vi "Welcome.vi"() -> ()   [LabVIEW 2017]
uses:
  Global/Global 1.vi
  Global/Login Details.vi
  Global/DATA LOG.vi
  Control/WELCOM SCREEN ENUM.ctl
panel:
  out "Screen Index":i32
  in  "Check 2":bool
  in  "auto":bool
  in  "Test Print":bool
  in  "andon":bool
  in  "MANUAL":bool
  out "error out 2":errorcluster
  in  "error in (no error) 3":errorcluster
  in  "Remove":bool
  in  "Check":bool
  in  "Home":bool
  out "user name":string
  out "STOP":bool
  in  "Tab Control":enum32{"Page 1", "user mangement"}(tab)
  out "error out":errorcluster
  in  "error in (no error)":errorcluster
  in  "LOGIN":bool
  in  "RECIPE":bool
  in  "EXIT":bool
  in  "REPORT":bool
  in  "Hardware Setting":bool
  in  "Shift Setting":bool
  in  "AUTO MODE":bool
  in  "USER MANGMENT":bool
  out "datetime":string
  # "PV Clean Mobility Technologies Traceability System"
  # "USER :"
  # "Powered By - NiVision Automation Systems Pvt. Ltd."
  # "Powered By-Infinity Automation Systems Pvt Ltd. Pune"
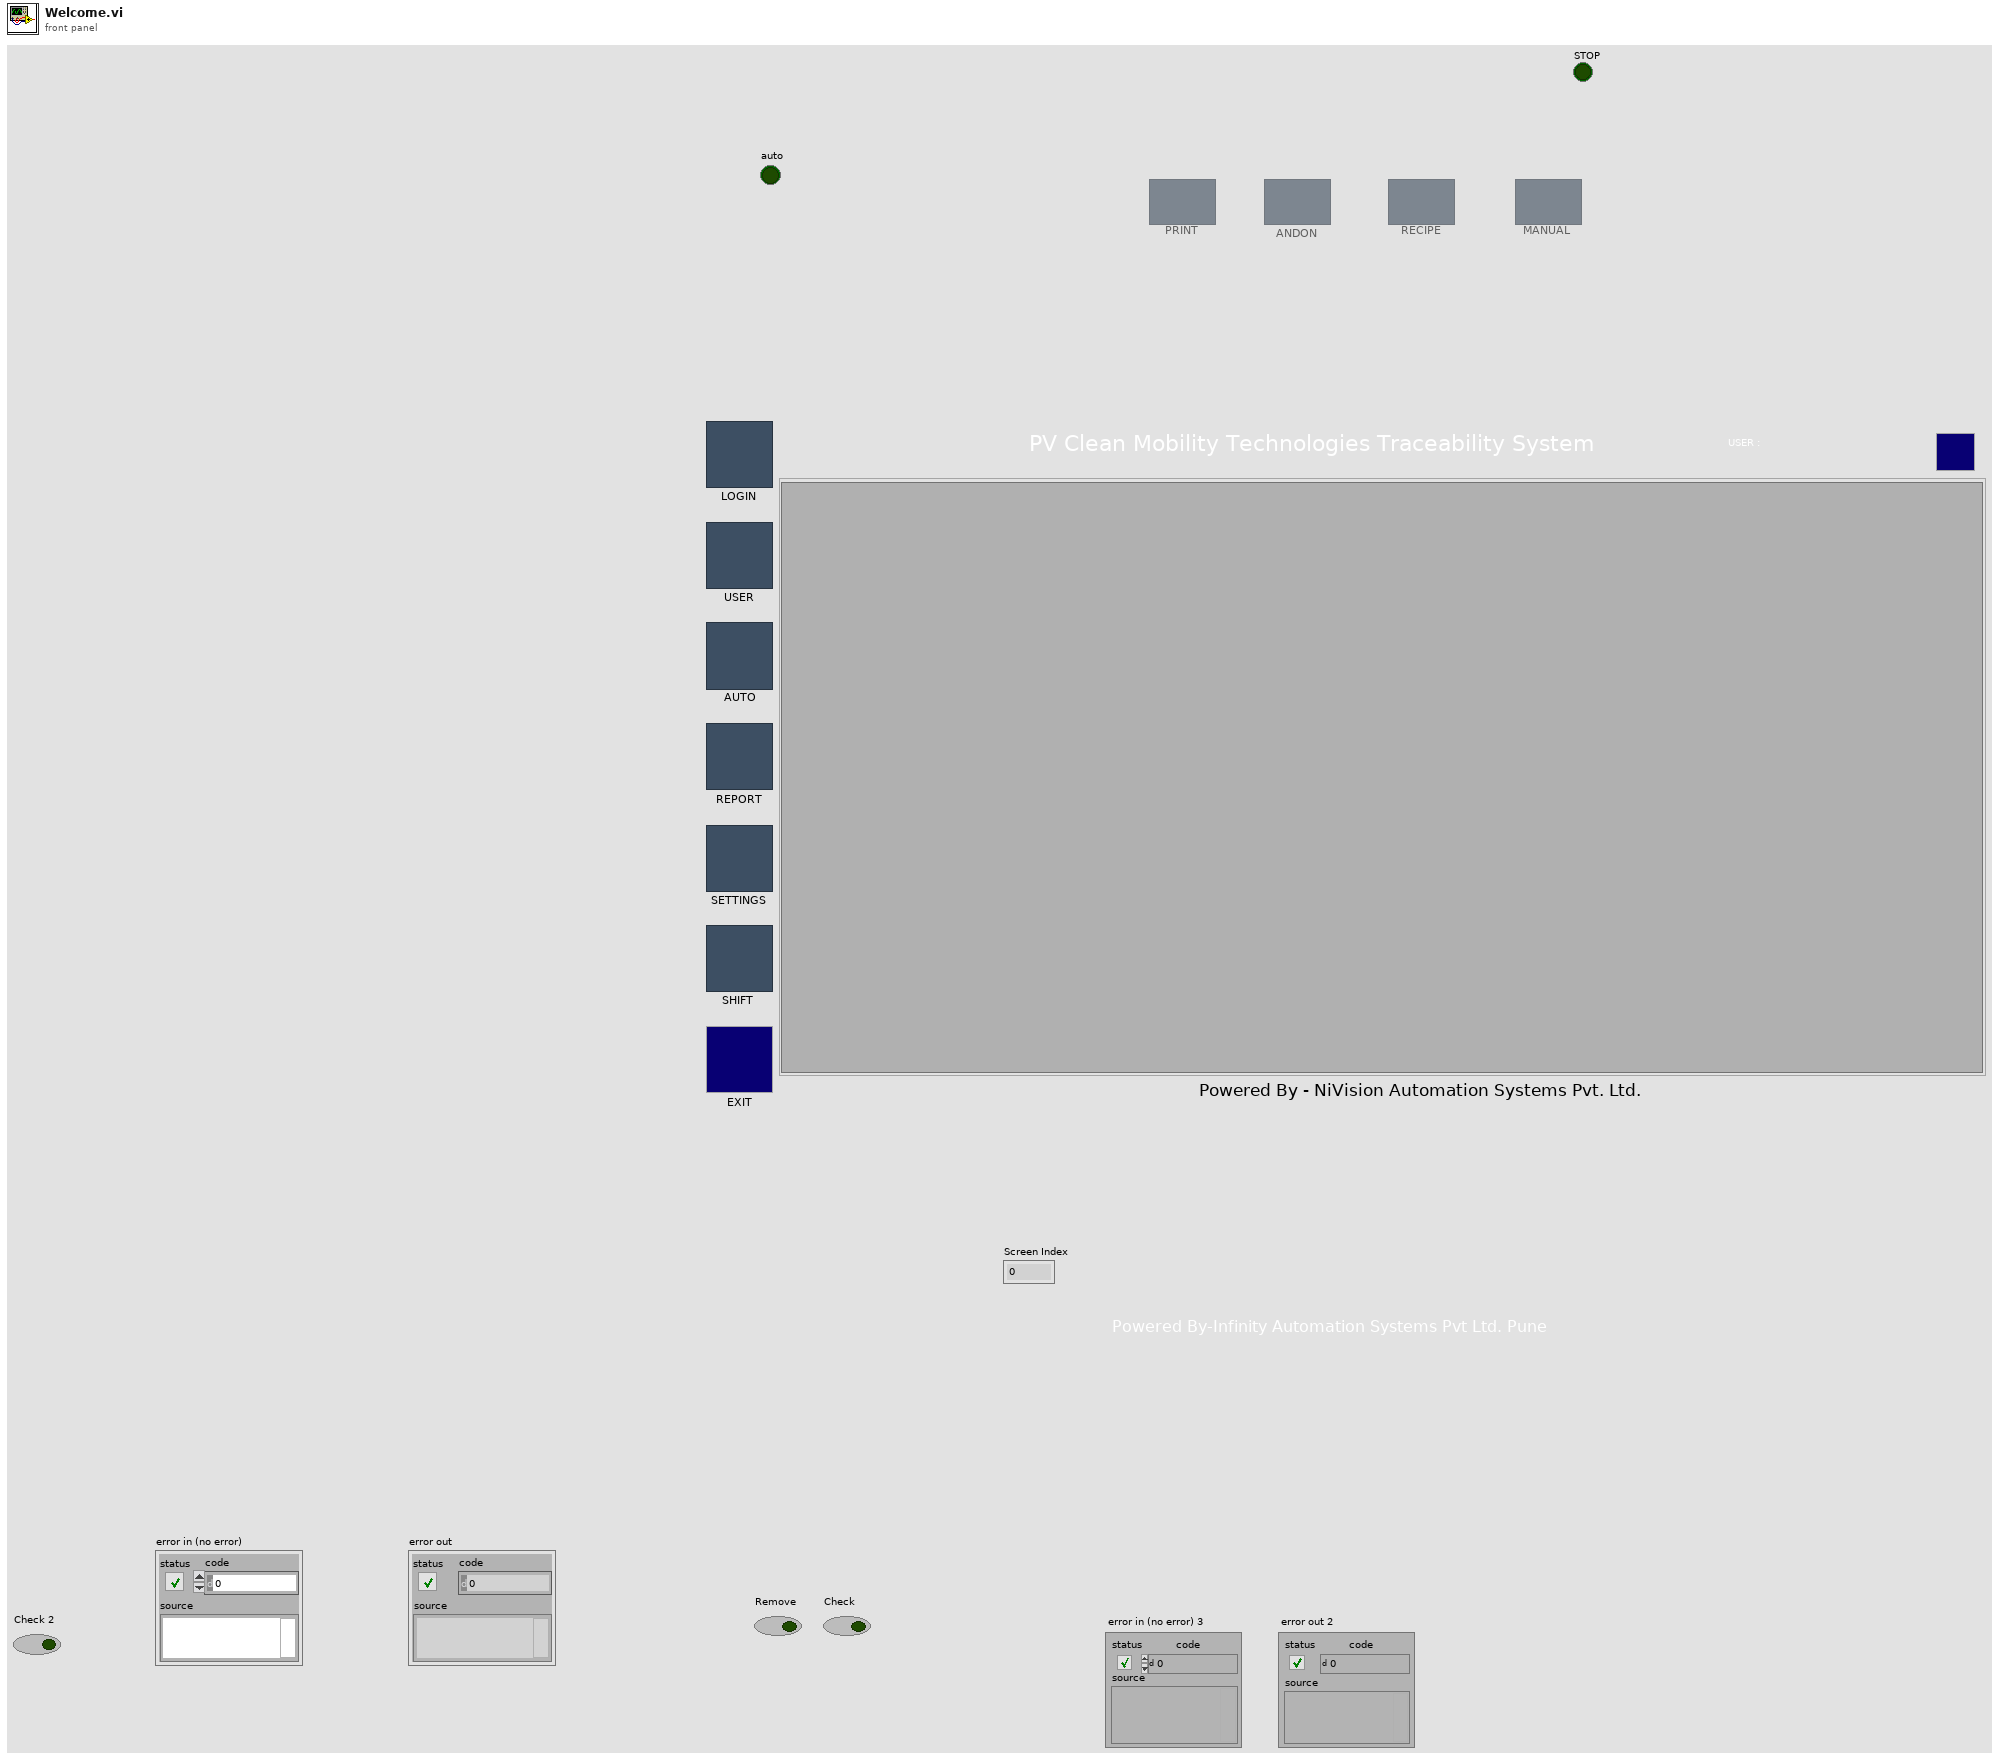
[diagram p1: front panel]
types:
  T1 = typedef "WELCOM SCREEN ENUM.ctl" = enum16{"Initialization", "Wait For Event", "RUN", "LOGIN", "USER MANAGEMENT", "AUTORITY MANAGEMENT", "AUTO MODE", "MANUAL MODE", "BIN MASTER", "CHEMICAL MASTER", "RAW MATERIAL INWARD", "RECIPE INGREDIENT", "REPORT", "SHIFT SETTING", "HARDWARE SETTING", "Check Authority", "TEST PRINT", "EXIT"}
  T2 = cluster{"SCREEN 1":bool, "SCREEN 2":bool, "SCREEN 3":bool, "SCREEN 4":bool, "SCREEN 5":bool, "SCREEN 6":bool, "SCREEN 7":bool, "SCREEN 8":bool, "SCREEN 9":bool, "SCREEN 10":bool, "SCREEN 11":bool, "SCREEN 12":bool, "SCREEN 13":bool, "SCREEN 14":bool, "SCREEN 15":bool, "SCREEN 16":bool, "SCREEN 17":bool, "SCREEN 18":bool, "SCREEN 19":bool, "SCREEN 20":bool}
  T3 = enum8{"Enabled", "Disabled", "Disabled and Grayed Out"}
  T4 = enum32{"Invalid", "Standard", "Closed", "Hidden", "Minimized", "Maximized"}
  T5 = enum32{"Bad", "Idle", "Run top level", "Running"}
  T6 = enum32{"invalid app kind", "Development System", "Run Time System", "Student Edition", "Embedded LabVIEW", "Evaluation", "Custom"}
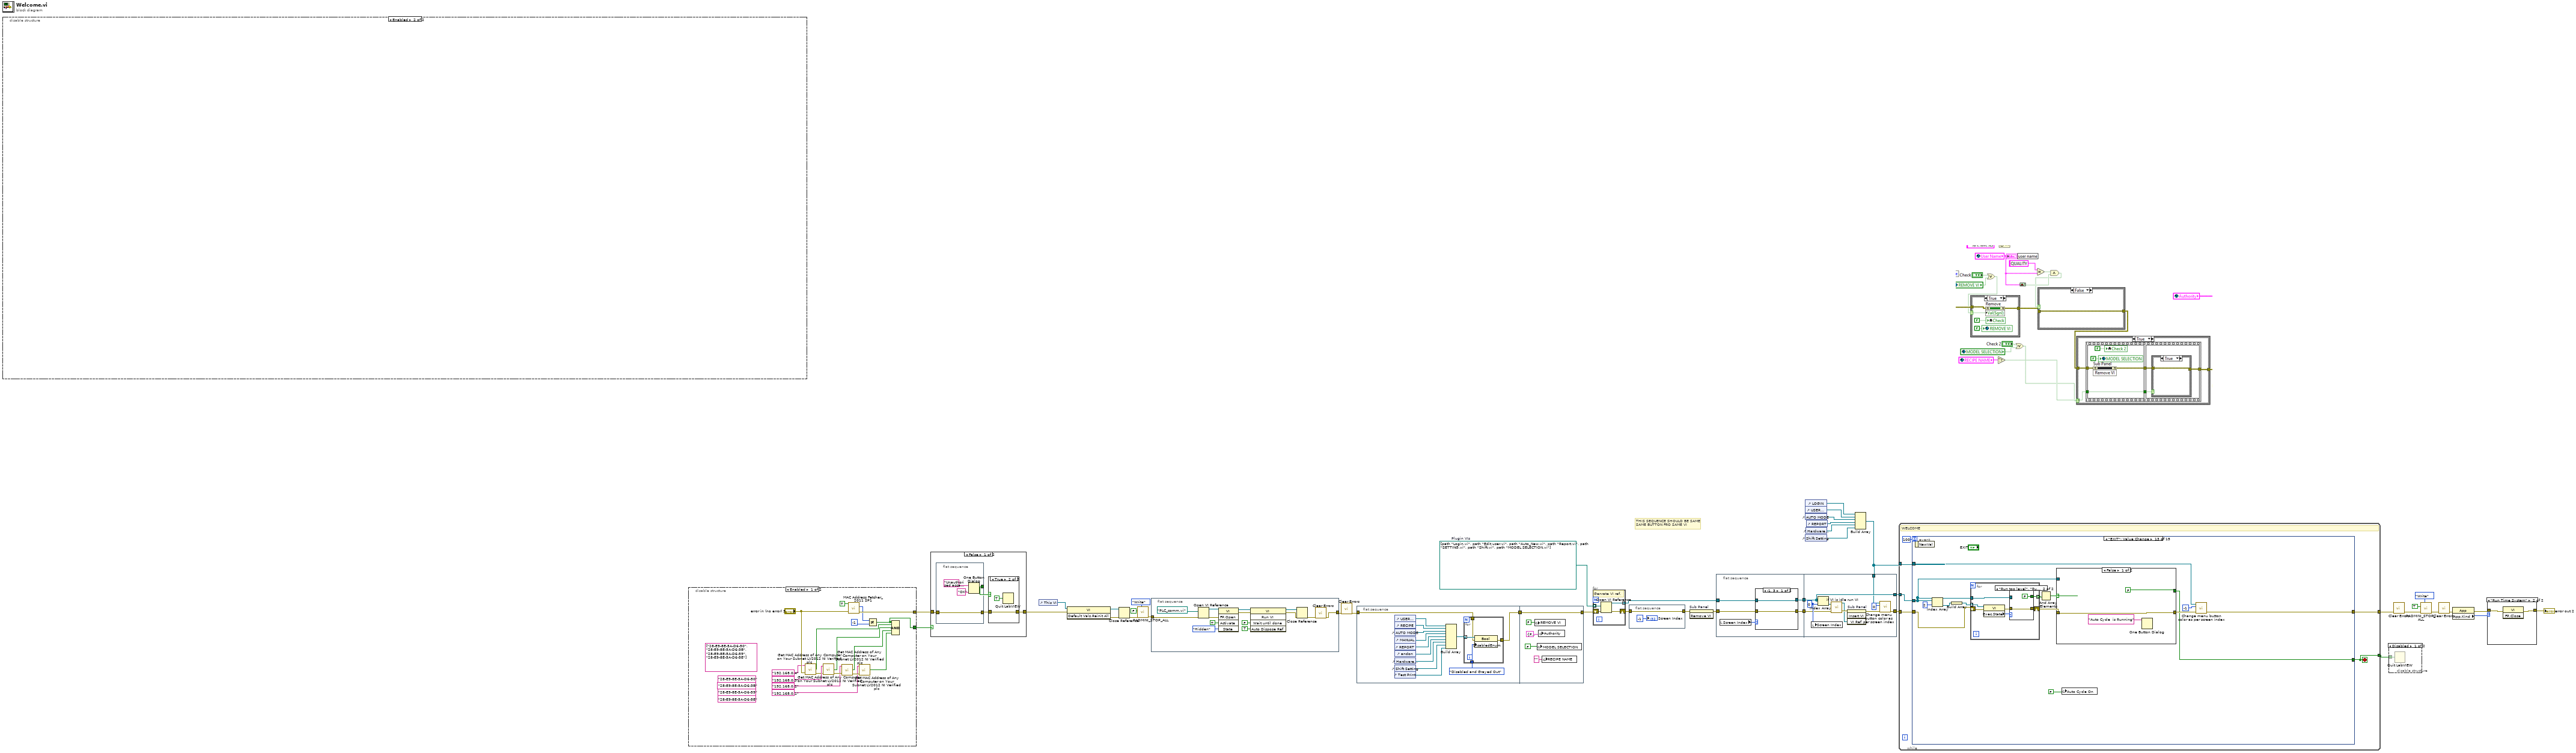
[diagram p0: block diagram]
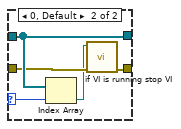
[diagram p2: hidden frame]
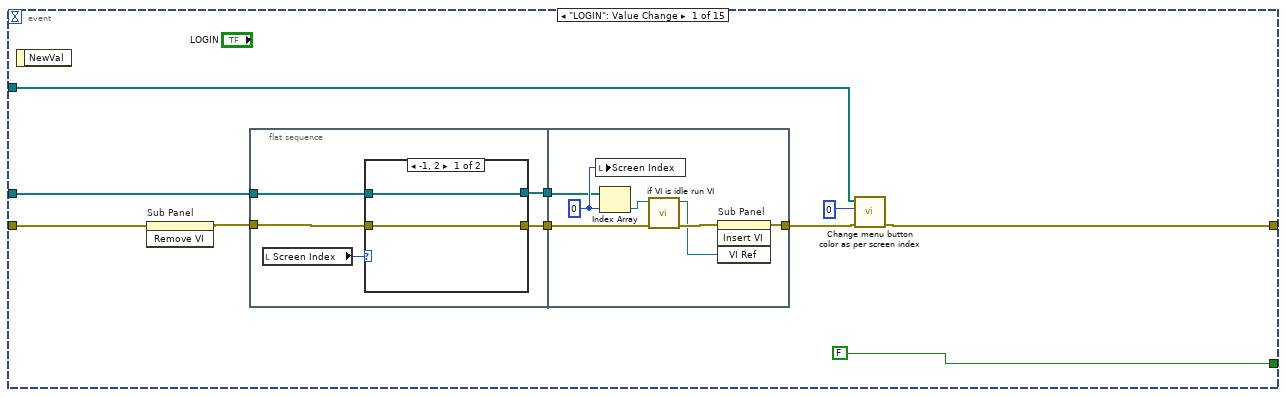
[diagram p5: hidden frame]
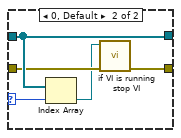
[diagram p6: hidden frame]
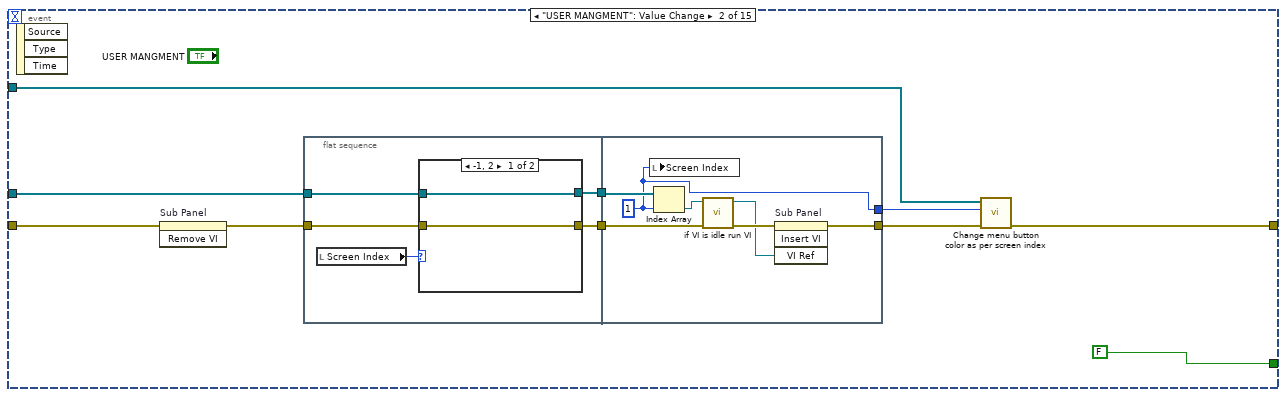
[diagram p7: hidden frame]
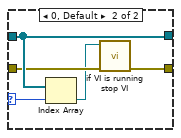
[diagram p8: hidden frame]
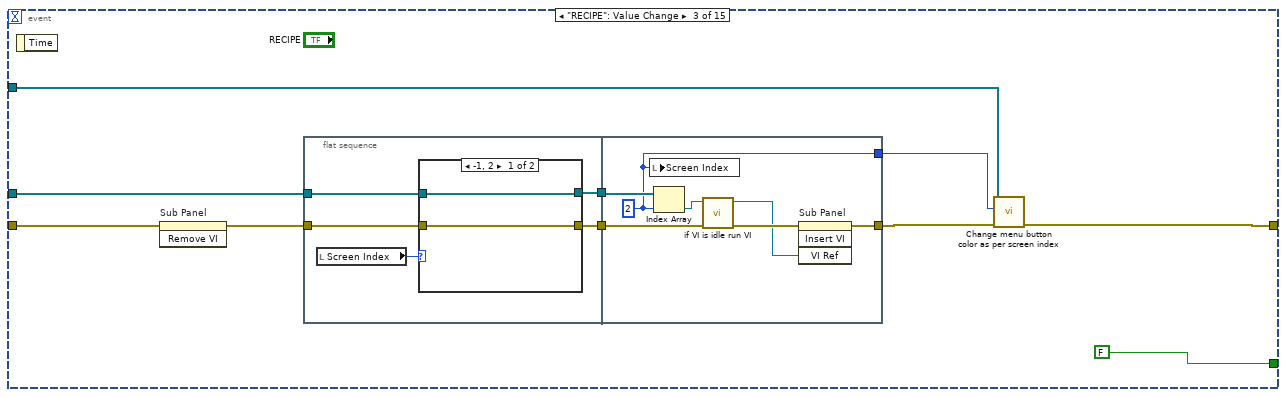
[diagram p9: hidden frame]
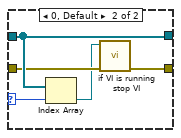
[diagram p10: hidden frame]
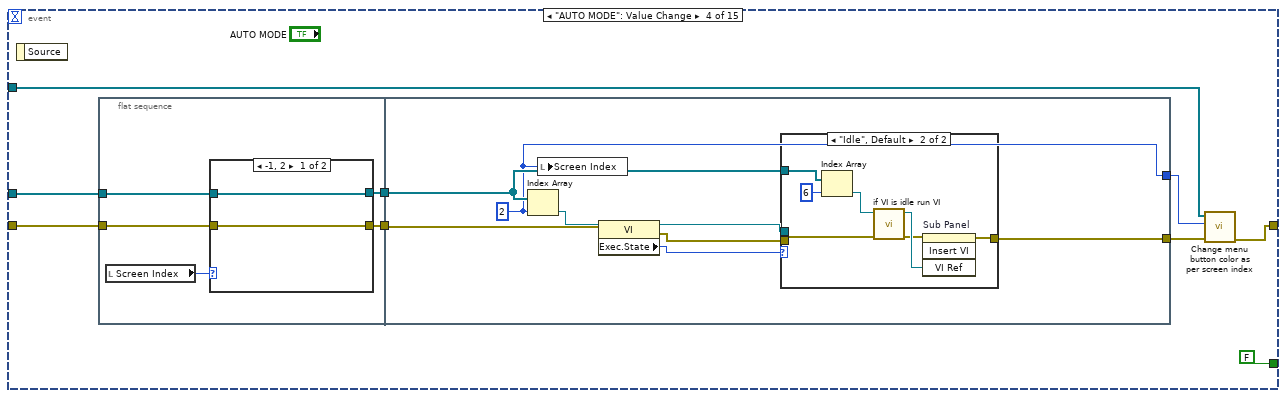
[diagram p11: hidden frame]
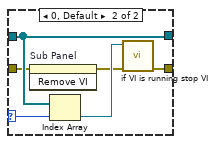
[diagram p12: hidden frame]
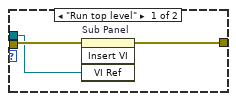
[diagram p13: hidden frame]
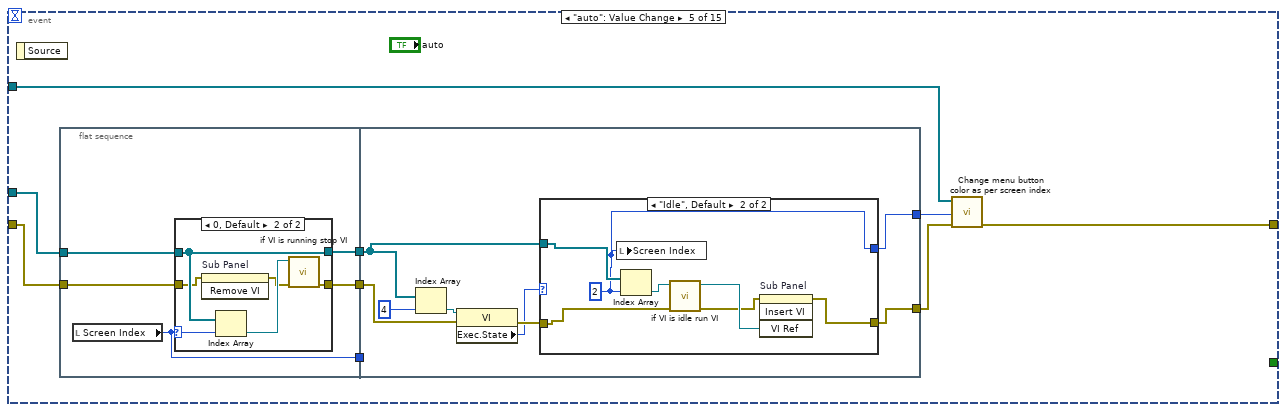
[diagram p14: hidden frame]
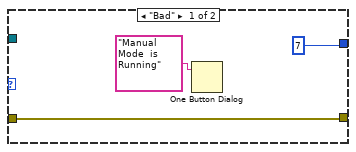
[diagram p16: hidden frame]
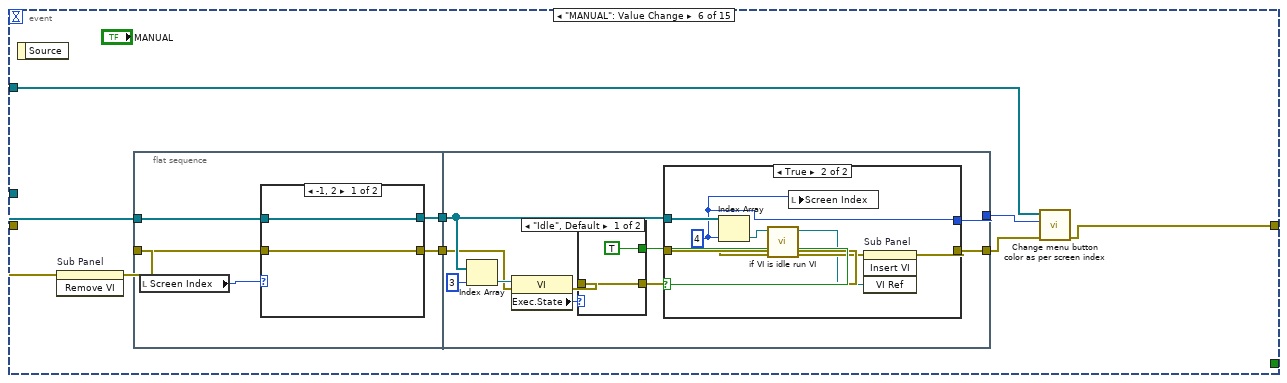
[diagram p17: hidden frame]
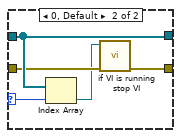
[diagram p18: hidden frame]
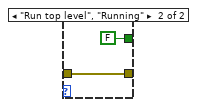
[diagram p19: hidden frame]
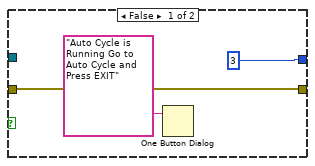
[diagram p20: hidden frame]
diagram:
  w33 = path[] [path "Login.vi", path "Edit user.vi", path "Auto_New.vi", path "Report.vi", path "SETTING.vi", path "Shift.vi", path "MODEL SELECTION.vi"]  # Plugin VIs
  # "THIS SEQUENCE SHOULD BE SAME\nSAME BUTTON FRO SAME VI"
  # "THIS SEQUENCE SHOULD BE SAME\nSAME BUTTON FRO SAME VI"
  n1 = disable-structure shown="Enabled" {
    frame Disabled {
      n2 = flat-sequence {
        tunnel: "error in (no error)" -> [w68]
        tunnel: [w67] -> w43
        frame #0 {
          n3 = invoke class="VI" method="Default Vals.Reinit All"(error in=w68) -> (error out=w67:errorcluster)  [unwired: 2 in, 2 out]
          n4 = global write "Login Details.vi" "Authority"(T2 {"SCREEN 1"=FALSE, "SCREEN 2"=FALSE, "SCREEN 3"=FALSE, "SCREEN 4"=FALSE, "SCREEN 5"=FALSE, "SCREEN 6"=FALSE, "SCREEN 7"=FALSE, "SCREEN 8"=FALSE, "SCREEN 9"=FALSE, "SCREEN 10"=FALSE, "SCREEN 11"=FALSE, "SCREEN 12"=FALSE, "SCREEN 13"=FALSE, "SCREEN 14"=FALSE, "SCREEN 15"=FALSE, "SCREEN 16"=FALSE, "SCREEN 17"=FALSE, "SCREEN 18"=FALSE, "SCREEN 19"=FALSE, "SCREEN 20"=FALSE} ("Authority")) -> ()
        }
      }
      n5 = invoke on="Sub Panel" class="SubPnl" method="Remove VI"(error in=w43) -> (error out=w56:errorcluster)  [unwired: 2 in, 2 out]
      n6 = Open VI Reference(vi path=path "Login.vi", error in (no error)=w56) -> (vi reference=w55:refnum<vi>, error out=w53:errorcluster)  [unwired: 4 in]
      n7 = invoke on="Sub Panel" class="SubPnl" method="Insert VI"(error in=w53, "VI Ref"=w55) -> (error out=w54:errorcluster)  [unwired: 2 in, 3 out]
      n8 = invoke class="VI" method="Run VI"(reference=w55, error in=w54, "Wait until done"=TRUE ("Wait Until Done"), "Auto Dispose Ref"=FALSE ("Auto Dispose Reference")) -> (reference out=w51:refnum<vi>, error out=w52:errorcluster)  [unwired: 1 in, 3 out]
      n9 = Close Reference(reference=w51, error in (no error)=w52) -> (error out=w46:errorcluster)
      n10 = Unbundle By Name(w46) -> ("code"=w50:i32)
      n11 = call <vilib>:"Clear Errors.vi"("error in (no error)"=w46) -> ("error out"=w48:errorcluster)  [unwired: 5 in, 1 out]
      n12 = Not Equal?(x=7, y=w50) -> (x != y?=w49:bool)
      n13 = Select(t=w46, s=w49, f=w48) -> (s? t:f=w47:errorcluster)
      n14 = call <vilib>:"Simple Error Handler.vi"("error in (no error)"=w47) -> ("error out"=w57:errorcluster)  [unwired: 4 in, 4 out]
      n15 = invoke on="Sub Panel" class="SubPnl" method="Remove VI"(error in=w57) -> (error out=w45:errorcluster)  [unwired: 2 in, 2 out]
      n16 = while {
        tunnel: w45 -> [w75]
        shift-right: [w77] -> _
        shift-left: WELCOM_SCREEN_ENUM."Initialization" -> [w71]
        shift-right: [w74] -> _
        shift-left: cluster{"VI Run":string} {"VI Run"=""} -> [w73]
        tunnel: [w76] -> w63
        stop <- w72 stop-if-true
        n17 = case shown="\"AUTORITY MANAGEMENT\"" w71 {
          tunnel: [WELCOM_SCREEN_ENUM."Check Authority" w102 WELCOM_SCREEN_ENUM."Wait For Event" WELCOM_SCREEN_ENUM."Wait For Event" WELCOM_SCREEN_ENUM."RUN" WELCOM_SCREEN_ENUM."RUN" WELCOM_SCREEN_ENUM."RUN" WELCOM_SCREEN_ENUM."RUN" WELCOM_SCREEN_ENUM."RUN" WELCOM_SCREEN_ENUM."RUN" WELCOM_SCREEN_ENUM."RUN" WELCOM_SCREEN_ENUM."RUN" WELCOM_SCREEN_ENUM."RUN" WELCOM_SCREEN_ENUM."RUN" WELCOM_SCREEN_ENUM."RUN" WELCOM_SCREEN_ENUM."RUN" WELCOM_SCREEN_ENUM."RUN" w229] -> w77
          tunnel: [w95 w101 w123 w127 w133 w139 w145 w151 w157 w163 w169 w175 w181 w187 w193 w199 w205 w224] -> w76
          tunnel: w75 -> [w95 w101 w123 w127 w133 w139 w145 w151 w157 w163 w169 w175 w181 w187 w193 w199 w205 w223]
          tunnel: [w93 w99 w122 w126 w131 w137 w142 w146 w155 w161 w167 w170 w177 w185 w188 w194 w203 w222] -> w74
          tunnel: w73 -> [w93 w99 w122 w126 w132 w138 w143 w147 w156 w162 w168 w171 w178 w186 w189 w195 w204 w222]
          tunnel: [FALSE FALSE FALSE TRUE FALSE FALSE FALSE FALSE FALSE FALSE FALSE FALSE FALSE FALSE FALSE FALSE FALSE FALSE] -> w72
          frame "Initialization", Default {
            n18 = control-ref of="USER MANGMENT"() -> (w80:refnum<vi>)
            n19 = control-ref of="RECIPE"() -> (w81:refnum<vi>)
            n20 = control-ref of="AUTO MODE"() -> (w82:refnum<vi>)
            n21 = control-ref of="REPORT"() -> (w88:refnum<vi>)
            n22 = control-ref of="Shift Setting"() -> (w89:refnum<vi>)
            n23 = control-ref of="Hardware Setting"() -> (w90:refnum<vi>)
            n24 = Build Array(w80, w81, w82, w88, w89, w90) -> (w79:refnum<vi>[], w83:refnum<vi>, w84:refnum<vi>, w85:refnum<vi>, w86:refnum<vi>, w87:refnum<vi>, w91:refnum<vi>)
            n25 = for {
              tunnel: w79 -> [w97] mode=indexing
              n26 = property class="Bool"(reference=w97, "DisabledEnum"=T3."Disabled and Grayed Out" ("Disabled")) -> ()  [unwired: 1 in, 2 out]
            }
          }
          frame "Wait For Event" {
            n27 = Search 1D Array(1D array=bool[] [], element=TRUE) -> (index of element=w104:i32)  [unwired: 1 in]
            n28 = case shown="11" w104 {
              tunnel: [WELCOM_SCREEN_ENUM."Wait For Event" WELCOM_SCREEN_ENUM."EXIT" WELCOM_SCREEN_ENUM."LOGIN" WELCOM_SCREEN_ENUM."USER MANAGEMENT" WELCOM_SCREEN_ENUM."AUTORITY MANAGEMENT" WELCOM_SCREEN_ENUM."AUTO MODE" WELCOM_SCREEN_ENUM."MANUAL MODE" WELCOM_SCREEN_ENUM."BIN MASTER" WELCOM_SCREEN_ENUM."CHEMICAL MASTER" WELCOM_SCREEN_ENUM."RAW MATERIAL INWARD" WELCOM_SCREEN_ENUM."REPORT" WELCOM_SCREEN_ENUM."SHIFT SETTING" WELCOM_SCREEN_ENUM."HARDWARE SETTING" WELCOM_SCREEN_ENUM."TEST PRINT" WELCOM_SCREEN_ENUM."RECIPE INGREDIENT"] -> w102
              frame -1, Default {
              }
              frame 0 {
              }
              frame 1 {
              }
              frame 2 {
              }
              frame 3 {
              }
              frame 4 {
              }
              frame 5 {
              }
              frame 6 {
              }
              frame 7 {
              }
              frame 8 {
              }
              frame 9 {
              }
              frame 10 {
              }
              frame 11 {
              }
              frame 12 {
              }
              frame 13 {
              }
            }
          }
          frame "Check Authority" {
          }
          frame "EXIT" {
          }
          frame "LOGIN" {
            w130 = "Login.vi"  # VI Run
            n29 = Bundle By Name(cluster=w132, "VI Run"=w130) -> (w131:cluster{"VI Run":string})
          }
          frame "USER MANAGEMENT" {
            w136 = "User Management.vi"  # VI Run
            n30 = Bundle By Name(cluster=w138, "VI Run"=w136) -> (w137:cluster{"VI Run":string})
          }
          frame "AUTORITY MANAGEMENT" {
            w141 = "Authority Management.vi"  # VI Run
            n31 = Bundle By Name(cluster=w143, "VI Run"=w141) -> (w142:cluster{"VI Run":string})
          }
          frame "AUTO MODE" {
            w148 = "AUTO MODE.vi"  # VI Run
            n32 = Bundle By Name(cluster=w147, "VI Run"=w148) -> (w146:cluster{"VI Run":string})
          }
          frame "MANUAL MODE" {
            w154 = "Manual Mode.vi"  # VI Run
            n33 = Bundle By Name(cluster=w156, "VI Run"=w154) -> (w155:cluster{"VI Run":string})
          }
          frame "BIN MASTER" {
            w160 = "Bin Master.vi"  # VI Run
            n34 = Bundle By Name(cluster=w162, "VI Run"=w160) -> (w161:cluster{"VI Run":string})
          }
          frame "CHEMICAL MASTER" {
            w166 = "Chemical Master.vi"  # VI Run
            n35 = Bundle By Name(cluster=w168, "VI Run"=w166) -> (w167:cluster{"VI Run":string})
          }
          frame "RAW MATERIAL INWARD" {
            w172 = "raw material inward.vi"  # VI Run
            n36 = Bundle By Name(cluster=w171, "VI Run"=w172) -> (w170:cluster{"VI Run":string})
          }
          frame "RECIPE INGREDIENT" {
            w179 = "Recipe_Ingredients.vi"  # VI Run
            n37 = Bundle By Name(cluster=w178, "VI Run"=w179) -> (w177:cluster{"VI Run":string})
          }
          frame "REPORT" {
            w184 = "Report.vi"  # VI Run
            n38 = Bundle By Name(cluster=w186, "VI Run"=w184) -> (w185:cluster{"VI Run":string})
          }
          frame "SHIFT SETTING" {
            w190 = "shift setting.vi"  # VI Run
            n39 = Bundle By Name(cluster=w189, "VI Run"=w190) -> (w188:cluster{"VI Run":string})
          }
          frame "HARDWARE SETTING" {
            w196 = "Hardware Setting.vi"  # VI Run
            n40 = Bundle By Name(cluster=w195, "VI Run"=w196) -> (w194:cluster{"VI Run":string})
          }
          frame "TEST PRINT" {
            w202 = "Test Print.vi"  # VI Run
            n41 = Bundle By Name(cluster=w204, "VI Run"=w202) -> (w203:cluster{"VI Run":string})
          }
          frame "RUN" {
            w230 = "Login.vi"  # x
            n42 = Unbundle By Name(w222) -> ("VI Run"=w231:string)
            n43 = invoke on="Sub Panel" class="SubPnl" method="Remove VI"(error in=w223) -> (error out=w212:errorcluster)  [unwired: 2 in, 2 out]
            n44 = Equal?(x=w230, y=w231) -> (x = y?=w228:bool)
            n45 = String To Path(string=w231) -> (path=w207:path)
            n46 = Open VI Reference(vi path=w207, error in (no error)=w212) -> (vi reference=w213:refnum<vi>, error out=w215:errorcluster)  [unwired: 4 in]
            n47 = invoke on="Sub Panel" class="SubPnl" method="Insert VI"(error in=w215, "VI Ref"=w213) -> (error out=w214:errorcluster)  [unwired: 2 in, 3 out]
            n48 = invoke class="VI" method="Run VI"(reference=w213, error in=w214, "Wait until done"=TRUE ("Wait Until Done"), "Auto Dispose Ref"=FALSE ("Auto Dispose Reference")) -> (reference out=w217:refnum<vi>, error out=w216:errorcluster)  [unwired: 1 in, 3 out]
            n49 = Close Reference(reference=w217, error in (no error)=w216) -> (error out=w206:errorcluster)
            n50 = Unbundle By Name(w206) -> ("code"=w218:i32)
            n51 = call <vilib>:"Clear Errors.vi"("error in (no error)"=w206) -> ("error out"=w220:errorcluster)  [unwired: 5 in, 1 out]
            n52 = Not Equal?(x=7, y=w218) -> (x != y?=w219:bool)
            n53 = Select(t=WELCOM_SCREEN_ENUM."Check Authority", s=w228, f=WELCOM_SCREEN_ENUM."Wait For Event") -> (s? t:f=w229:T1)
            n54 = Select(t=w206, s=w219, f=w220) -> (s? t:f=w221:errorcluster)
            n55 = call <vilib>:"Simple Error Handler.vi"("error in (no error)"=w221) -> ("error out"=w211:errorcluster)  [unwired: 4 in, 4 out]
            n56 = invoke on="Sub Panel" class="SubPnl" method="Remove VI"(error in=w211) -> (error out=w224:errorcluster)  [unwired: 2 in, 2 out]
          }
        }
        "STOP" <- w72
        n57 = Wait (ms)(milliseconds to wait=u32 100) -> ()  [unwired: 1 out]
      }
      n58 = while {
        tunnel: w43 -> [w65]
        tunnel: [w65] -> w41
        stop <- w66 stop-if-true
        n59 = local read "STOP"() -> (w66:bool)
      }
      n60 = Merge Errors(w41, w63) -> (→"error out":errorcluster)
      n61 = disable-structure shown="Enabled" {
        disable-tunnel: w63 -> [w70 _]
        frame Enabled {
          n62 = invoke class="VI" method="FP.Close"(error in=w70) -> ()  [unwired: 2 in, 3 out]
        }
        frame Disabled {
        }
      }
    }
    frame Enabled {
    }
  }
  n63 = disable-structure shown="Enabled" {
    disable-tunnel: [w247 _] -> w5
    disable-tunnel: [w232 TRUE] -> w1
    frame Enabled {
      (unwired) string[] ["28-E9-8E-5A-D6-50", "28-E9-8E-5A-D6-3B", "28-E9-8E-5A-D6-59", "28-E9-8E-5A-D6-5E"]
      (unwired) "28-E9-8E-5A-D6-5E" ("IP Address")
      (unwired) "28-E9-8E-5A-D6-59" ("IP Address")
      (unwired) "28-E9-8E-5A-D6-3B" ("IP Address")
      (unwired) "28-E9-8E-5A-D6-50" ("IP Address")
      n64 = call "Get MAC Address of Any Computer on Your Subnet LV2012 NI Verified plc.vi"("error constant"="error in (no error) 3", "IP Address"="192.168.0.4") -> ("error out"=w243:errorcluster, "x .and. y?"=w236:bool)  [unwired: 1 in, 1 out]
      n65 = call "Get MAC Address of Any Computer on Your Subnet LV2012 NI Verified plc.vi"("error constant"=w243, "IP Address"="192.168.0.3") -> ("error out"=w241:errorcluster, "x .and. y?"=w235:bool)  [unwired: 1 in, 1 out]
      n66 = call "Get MAC Address of Any Computer on Your Subnet LV2012 NI Verified plc.vi"("error constant"=w241, "IP Address"="192.168.0.2") -> ("error out"=w242:errorcluster, "x .and. y?"=w234:bool)  [unwired: 1 in, 1 out]
      n67 = call "MAC Address Fetcher_2011 SP1.vi"("error in (no error)"="error in (no error) 3", "Search all adapters?"=TRUE) -> ("error out"=w247:errorcluster, "index of element"=w238:i32)  [unwired: 6 in, 2 out]
      n68 = call "Get MAC Address of Any Computer on Your Subnet LV2012 NI Verified plc.vi"("error constant"=w242, "IP Address"="192.168.0.1") -> ("x .and. y?"=w233:bool)  [unwired: 1 in, 2 out]
      n69 = Not Equal?(x=w238, y=-1) -> (x != y?=w232:bool)
      n70 = Compound Arithmetic op=AND(w232, w236, w235, w234, w233) -> ()  [unwired: 1 out]
    }
    frame Disabled {
    }
  }
  n71 = case shown="False" w1 {
    tunnel: w5 -> [w251 w261]
    tunnel: [w250 w261] -> w4
    frame False {
      n72 = flat-sequence {
        tunnel: [w256] -> w253
        tunnel: [w255] -> w252
        tunnel: w251 -> [w255]
        frame #0 {
          n73 = One Button Dialog(message="Unauthorised access to this system\nPlease contact to NIVision Automation Systems Pvt Ltd", button name ("OK")="OK") -> (true=w256:bool)
        }
      }
      n74 = case shown="True" w253 {
        tunnel: w252 -> [w258 w259]
        tunnel: [w258 w259] -> w250
        frame False {
        }
        frame True {
          n75 = Quit LabVIEW(quit? (T)=TRUE) -> ()
        }
      }
    }
    frame True {
    }
  }
  n76 = control-ref of="This VI"() -> (w40:refnum<vi>)
  n77 = invoke class="VI" method="Default Vals.Reinit All"(reference=w40, error in=w4) -> (reference out=w38:refnum<vi>, error out=w39:errorcluster)  [unwired: 1 in, 1 out]
  n78 = Close Reference(reference=w38, error in (no error)=w39) -> (error out=w2:errorcluster)
  n79 = call "PADMINI_STOP_ALL.vi"("Enum"=enum16{"Read", "Write"}."Write", "error in (no error)"=w2, "Boolean"=FALSE) -> ("error out"=w6:errorcluster)  [unwired: 7 in, 1 out]
  n80 = flat-sequence {
    tunnel: w6 -> [w275]
    tunnel: [w273] -> w21
    frame #0 {
      n81 = Open VI Reference(vi path=path "PLC_comm.vi", error in (no error)=w275) -> (vi reference=w266:refnum<vi>, error out=w267:errorcluster)  [unwired: 4 in]
      n82 = invoke class="VI" method="FP.Open"(reference=w266, error in=w267, "Activate"=TRUE ("Activate?"), "State"=T4."Hidden") -> (reference out=w269:refnum<vi>, error out=w268:errorcluster)  [unwired: 1 in, 3 out]
      n83 = invoke class="VI" method="Run VI"(reference=w269, error in=w268, "Wait until done"=FALSE ("Wait Until Done"), "Auto Dispose Ref"=TRUE ("Auto Dispose Reference")) -> (reference out=w264:refnum<vi>, error out=w263:errorcluster)  [unwired: 1 in, 3 out]
      n84 = Close Reference(reference=w264, error in (no error)=w263) -> (error out=w274:errorcluster)
      n85 = call <vilib>:"Clear Errors.vi"("error in (no error)"=w274) -> ("error out"=w273:errorcluster)  [unwired: 5 in, 1 out]
    }
  }
  n86 = call <vilib>:"Clear Errors.vi"("error in (no error)"=w21) -> ("error out"=w20:errorcluster)  [unwired: 5 in, 1 out]
  n87 = flat-sequence {
    tunnel: w20 -> [w277]
    tunnel: [w276] -> w13
    tunnel: [w297] -> w23
    tunnel: w13 -> [w297]
    frame #0 {
      n88 = control-ref of="Shift Setting"() -> (w281:refnum<vi>)
      n89 = control-ref of="Test Print"() -> (w280:refnum<vi>)
      n90 = control-ref of="USER MANGMENT"() -> (w288:refnum<vi>)
      n91 = control-ref of="RECIPE"() -> (w287:refnum<vi>)
      n92 = control-ref of="AUTO MODE"() -> (w286:refnum<vi>)
      n93 = control-ref of="MANUAL"() -> (w285:refnum<vi>)
      n94 = control-ref of="REPORT"() -> (w284:refnum<vi>)
      n95 = control-ref of="andon"() -> (w283:refnum<vi>)
      n96 = control-ref of="Hardware Setting"() -> (w282:refnum<vi>)
      n97 = Build Array(w288, w287, w286, w285, w284, w283, w282, w281, w280) -> (w279:refnum<vi>[])
      n98 = for {
        tunnel: w279 -> [w292] mode=indexing
        tunnel: w277 -> [w291]
        tunnel: T3."Disabled and Grayed Out" ("Disabled") -> [w290]
        tunnel: [w289] -> w276
        n99 = property class="Bool"(reference=w292, error in=w291, "DisabledEnum"=w290) -> (error out=w289:errorcluster)  [unwired: 1 out]
      }
    }
    frame #1 {
      n100 = global write "Global 1.vi" "REMOVE VI"(FALSE ("REMOVE VI")) -> ()
      n101 = global write "Global 1.vi" "MODEL SELECTION"(FALSE ("REMOVE VI")) -> ()
      n102 = global write "Login Details.vi" "Authority"(T2 {"SCREEN 1"=FALSE, "SCREEN 2"=FALSE, "SCREEN 3"=FALSE, "SCREEN 4"=FALSE, "SCREEN 5"=FALSE, "SCREEN 6"=FALSE, "SCREEN 7"=FALSE, "SCREEN 8"=FALSE, "SCREEN 9"=FALSE, "SCREEN 10"=FALSE, "SCREEN 11"=FALSE, "SCREEN 12"=FALSE, "SCREEN 13"=FALSE, "SCREEN 14"=FALSE, "SCREEN 15"=FALSE, "SCREEN 16"=FALSE, "SCREEN 17"=FALSE, "SCREEN 18"=FALSE, "SCREEN 19"=FALSE, "SCREEN 20"=FALSE} ("Authority")) -> ()
      n103 = global write "Global 1.vi" "RECIPE NAME"("" ("RECIPE NAME")) -> ()
    }
  }
  n104 = for {
    tunnel: w33 -> [w299] mode=indexing
    tunnel: [w300] -> w26 mode=indexing
    shift-right: [w301] -> w32
    shift-left: w23 -> [w298]
    # "Genrate VI ref."
    n105 = Open VI Reference(vi path=w299, error in (no error)=w298) -> (vi reference=w300:refnum<vi>, error out=w301:errorcluster)  [unwired: 4 in]
  }
  n106 = flat-sequence {
    tunnel: w32 -> [w303]
    tunnel: [w303] -> w28
    frame #0 {
      "Screen Index" <- -1 ("Screen Index")
    }
  }
  n107 = invoke on="Sub Panel" class="SubPnl" method="Remove VI"(error in=w28) -> (error out=w29:errorcluster)  [unwired: 2 in, 2 out]
  n108 = flat-sequence {
    tunnel: w26 -> [w306]
    tunnel: [w308] -> w31
    tunnel: [w305] -> w30
    tunnel: w29 -> [w304]
    tunnel: w31 -> [w324]
    tunnel: w30 -> [w320]
    tunnel: [w317] -> w27
    tunnel: [w320] -> w25
    tunnel: w24 -> [w316]
    frame #0 {
      n109 = local read "Screen Index"() -> (w307:i32)
      n110 = case shown="-1, 3" w307 {
        selector: w307 -> [_ w315]
        tunnel: w304 -> [w310 w313]
        tunnel: [w310 w312] -> w308
        tunnel: w306 -> [w309 w314]
        tunnel: [w309 w314] -> w305
        frame -1, 3 {
        }
        frame 0, Default {
          n111 = Index Array(array=w314, index=w315) -> (element=w311:refnum<vi>)
          n112 = call "if VI is running stop VI.vi"("error in (no error)"=w313, "VI in"=w311) -> ("error out"=w312:errorcluster)  [unwired: 8 in, 1 out]
        }
      }
    }
    frame #1 {
      w325 = 0 ("index")
      n113 = local write "Screen Index"(w325) -> ()
      n114 = Index Array(array=w320, index=w325) -> (element=w323:refnum<vi>)
      n115 = call "if VI is idle run VI.vi"("error in (no error)"=w324, "VI in"=w323) -> ("error out"=w322:errorcluster, "VI out"=w321:refnum<vi>)  [unwired: 8 in]
      n116 = invoke on="Sub Panel" class="SubPnl" method="Insert VI"(error in=w322, "VI Ref"=w321) -> (error out=w318:errorcluster)  [unwired: 2 in, 3 out]
      n117 = call "Change menu button color as per screen index.vi"("error in (no error)"=w318, "Screen Index"=0, "Array"=w316) -> ("error out"=w317:errorcluster)  [unwired: 8 in]
    }
  }
  n118 = control-ref of="LOGIN"() -> (w19:refnum<vi>)
  n119 = control-ref of="USER MANGMENT"() -> (w18:refnum<vi>)
  n120 = control-ref of="AUTO MODE"() -> (w17:refnum<vi>)
  n121 = control-ref of="Shift Setting"() -> (w14:refnum<vi>)
  n122 = control-ref of="Hardware Setting"() -> (w15:refnum<vi>)
  n123 = control-ref of="REPORT"() -> (w16:refnum<vi>)
  n124 = Build Array(w19, w18, w17, w16, w15, w14) -> (w24:refnum<vi>[])
  n125 = while {
    tunnel: w27 -> [w328]
    tunnel: [w330] -> w22
    tunnel: w25 -> [w327]
    tunnel: w24 -> [w329]
    tunnel: [w326] -> w3
    stop <- w326 stop-if-true
    # "WELCOME"
    n126 = event shown="[12] \"EXIT\": Value Change" {
      selector: _ -> [_ _ _ _ _ _ _ _ _ _ _ _ _ _ _]
      dyn-events: _ -> [_ _ _ _ _ _ _ _ _ _ _ _ _ _ _]
      timeout: 100 -> [_ _ _ _ _ _ _ _ _ _ _ _ _ _ _]
      tunnel: [FALSE FALSE FALSE FALSE _ _ FALSE FALSE FALSE FALSE FALSE FALSE w697 FALSE FALSE] -> w326
      tunnel: [w334 w365 w394 w426 w459 w499 w548 w577 w606 w635 w664 w691 w696 w737 w740] -> w330
      tunnel: w327 -> [w340 w369 w398 w422 w463 w502 w552 w581 w610 w639 w668 _ w698 _ _]
      tunnel: w329 -> [w333 w363 w391 w425 w462 w500 w546 w574 w603 w633 w661 w690 w701 w735 _]
      tunnel: w328 -> [w332 w361 w390 w421 w464 w501 w544 w573 w602 w631 w660 w689 w705 w734 w752]
      event "LOGIN": Value Change {
        n127 = event-data() -> ()  [unwired: 1 in, 1 out]
        n128 = invoke on="Sub Panel" class="SubPnl" method="Remove VI"(error in=w332) -> (error out=w337:errorcluster)  [unwired: 2 in, 2 out]
        n129 = flat-sequence {
          tunnel: w340 -> [w344]
          tunnel: [w346] -> w339
          tunnel: [w343] -> w338
          tunnel: w337 -> [w342]
          tunnel: w339 -> [w358]
          tunnel: w338 -> [w359]
          tunnel: [w354] -> w335
          frame #0 {
            n130 = local read "Screen Index"() -> (w345:i32)
            n131 = case shown="-1, 2" w345 {
              selector: w345 -> [_ w353]
              tunnel: w342 -> [w348 w351]
              tunnel: [w348 w350] -> w346
              tunnel: w344 -> [w347 w352]
              tunnel: [w347 w352] -> w343
              frame -1, 2 {
              }
              frame 0, Default {
                n132 = Index Array(array=w352, index=w353) -> (element=w349:refnum<vi>)
                n133 = call "if VI is running stop VI.vi"("error in (no error)"=w351, "VI in"=w349) -> ("error out"=w350:errorcluster)  [unwired: 8 in, 1 out]
              }
            }
          }
          frame #1 {
            w360 = 0 ("index")
            n134 = local write "Screen Index"(w360) -> ()
            n135 = Index Array(array=w359, index=w360) -> (element=w357:refnum<vi>)
            n136 = call "if VI is idle run VI.vi"("error in (no error)"=w358, "VI in"=w357) -> ("error out"=w356:errorcluster, "VI out"=w355:refnum<vi>)  [unwired: 8 in]
            n137 = invoke on="Sub Panel" class="SubPnl" method="Insert VI"(error in=w356, "VI Ref"=w355) -> (error out=w354:errorcluster)  [unwired: 2 in, 3 out]
          }
        }
        n138 = call "Change menu button color as per screen index.vi"("error in (no error)"=w335, "Screen Index"=0, "Array"=w333) -> ("error out"=w334:errorcluster)  [unwired: 8 in]
      }
      event "USER MANGMENT": Value Change {
        n139 = event-data() -> ()  [unwired: 1 in, 3 out]
        n140 = invoke on="Sub Panel" class="SubPnl" method="Remove VI"(error in=w361) -> (error out=w366:errorcluster)  [unwired: 2 in, 2 out]
        n141 = flat-sequence {
          tunnel: w366 -> [w375]
          tunnel: w369 -> [w372]
          tunnel: [w374] -> w368
          tunnel: [w371] -> w367
          tunnel: [w388] -> w364
          tunnel: w368 -> [w387]
          tunnel: w367 -> [w389]
          tunnel: [w383] -> w362
          frame #0 {
            n142 = local read "Screen Index"() -> (w373:i32)
            n143 = case shown="-1, 2" w373 {
              selector: w373 -> [_ w382]
              tunnel: w375 -> [w377 w380]
              tunnel: [w377 w379] -> w374
              tunnel: w372 -> [w376 w381]
              tunnel: [w376 w381] -> w371
              frame -1, 2 {
              }
              frame 0, Default {
                n144 = Index Array(array=w381, index=w382) -> (element=w378:refnum<vi>)
                n145 = call "if VI is running stop VI.vi"("error in (no error)"=w380, "VI in"=w378) -> ("error out"=w379:errorcluster)  [unwired: 8 in, 1 out]
              }
            }
          }
          frame #1 {
            w383 = 1 ("index")
            n146 = local write "Screen Index"(w383) -> ()
            n147 = Index Array(array=w389, index=w383) -> (element=w385:refnum<vi>)
            n148 = call "if VI is idle run VI.vi"("error in (no error)"=w387, "VI in"=w385) -> ("error out"=w386:errorcluster, "VI out"=w384:refnum<vi>)  [unwired: 8 in]
            n149 = invoke on="Sub Panel" class="SubPnl" method="Insert VI"(error in=w386, "VI Ref"=w384) -> (error out=w388:errorcluster)  [unwired: 2 in, 3 out]
          }
        }
        n150 = call "Change menu button color as per screen index.vi"("error in (no error)"=w364, "Screen Index"=w362, "Array"=w363) -> ("error out"=w365:errorcluster)  [unwired: 8 in]
      }
      event "RECIPE": Value Change {
        n151 = event-data() -> ()  [unwired: 1 in, 1 out]
        n152 = invoke on="Sub Panel" class="SubPnl" method="Remove VI"(error in=w390) -> (error out=w395:errorcluster)  [unwired: 2 in, 2 out]
        n153 = flat-sequence {
          tunnel: w395 -> [w404]
          tunnel: w398 -> [w401]
          tunnel: [w403] -> w397
          tunnel: [w400] -> w396
          tunnel: [w417] -> w393
          tunnel: w397 -> [w416]
          tunnel: w396 -> [w418]
          tunnel: [w412] -> w392
          frame #0 {
            n154 = local read "Screen Index"() -> (w402:i32)
            n155 = case shown="-1, 2" w402 {
              selector: w402 -> [_ w411]
              tunnel: w404 -> [w406 w409]
              tunnel: [w406 w408] -> w403
              tunnel: w401 -> [w405 w410]
              tunnel: [w405 w410] -> w400
              frame -1, 2 {
              }
              frame 0, Default {
                n156 = Index Array(array=w410, index=w411) -> (element=w407:refnum<vi>)
                n157 = call "if VI is running stop VI.vi"("error in (no error)"=w409, "VI in"=w407) -> ("error out"=w408:errorcluster)  [unwired: 8 in, 1 out]
              }
            }
          }
          frame #1 {
            w412 = 2 ("index")
            n158 = local write "Screen Index"(w412) -> ()
            n159 = Index Array(array=w418, index=w412) -> (element=w413:refnum<vi>)
            n160 = call "if VI is idle run VI.vi"("error in (no error)"=w416, "VI in"=w413) -> ("error out"=w415:errorcluster, "VI out"=w414:refnum<vi>)  [unwired: 8 in]
            n161 = invoke on="Sub Panel" class="SubPnl" method="Insert VI"(error in=w415, "VI Ref"=w414) -> (error out=w417:errorcluster)  [unwired: 2 in, 3 out]
          }
        }
        n162 = call "Change menu button color as per screen index.vi"("error in (no error)"=w393, "Screen Index"=w392, "Array"=w391) -> ("error out"=w394:errorcluster)  [unwired: 8 in]
      }
      event "AUTO MODE": Value Change {
        n163 = event-data() -> ()  [unwired: 1 in, 1 out]
        n164 = flat-sequence {
          tunnel: w421 -> [w432]
          tunnel: w422 -> [w430]
          tunnel: [w431] -> w424
          tunnel: [w429] -> w423
          tunnel: [w445] -> w419
          tunnel: w424 -> [w448]
          tunnel: w423 -> [w447]
          tunnel: [w446] -> w420
          frame #0 {
            n165 = local read "Screen Index"() -> (w428:i32)
            n166 = case shown="-1, 2" w428 {
              selector: w428 -> [_ w440]
              tunnel: w432 -> [w434 w436]
              tunnel: [w434 w438] -> w431
              tunnel: w430 -> [w433 w439]
              tunnel: [w433 w439] -> w429
              frame -1, 2 {
              }
              frame 0, Default {
                n167 = invoke on="Sub Panel" class="SubPnl" method="Remove VI"(error in=w436) -> (error out=w435:errorcluster)  [unwired: 2 in, 2 out]
                n168 = Index Array(array=w439, index=w440) -> (element=w437:refnum<vi>)
                n169 = call "if VI is running stop VI.vi"("error in (no error)"=w435, "VI in"=w437) -> ("error out"=w438:errorcluster)  [unwired: 8 in, 1 out]
              }
            }
          }
          frame #1 {
            w446 = 2 ("index")
            n170 = Index Array(array=w447, index=w446) -> (element=w441:refnum<vi>)
            n171 = local write "Screen Index"(w446) -> ()
            n172 = property class="VI"(reference=w441, error in=w448) -> (reference out=w442:refnum<vi>, error out=w443:errorcluster, "Exec.State"=w444:T5)
            n173 = case shown="\"Idle\", Default" w444 {
              tunnel: [w451 w456] -> w445
              tunnel: w443 -> [w450 w457]
              tunnel: w442 -> [w449 _]
              tunnel: w447 -> [_ w455]
              frame "Run top level" {
                n174 = invoke on="Sub Panel" class="SubPnl" method="Insert VI"(error in=w450, "VI Ref"=w449) -> (error out=w451:errorcluster)  [unwired: 2 in, 3 out]
              }
              frame "Idle", Default {
                n175 = Index Array(array=w455, index=6) -> (element=w454:refnum<vi>)
                n176 = call "if VI is idle run VI.vi"("error in (no error)"=w457, "VI in"=w454) -> ("error out"=w452:errorcluster, "VI out"=w458:refnum<vi>)  [unwired: 8 in]
                n177 = invoke on="Sub Panel" class="SubPnl" method="Insert VI"(error in=w452, "VI Ref"=w458) -> (error out=w456:errorcluster)  [unwired: 2 in, 3 out]
              }
            }
          }
        }
        n178 = call "Change menu button color as per screen index.vi"("error in (no error)"=w419, "Screen Index"=w420, "Array"=w425) -> ("error out"=w426:errorcluster)  [unwired: 8 in]
      }
      event "auto": Value Change {
        n179 = event-data() -> ()  [unwired: 1 in, 1 out]
        n180 = flat-sequence {
          tunnel: w464 -> [w472]
          tunnel: w463 -> [w470]
          tunnel: [w471] -> w467
          tunnel: [w469] -> w466
          tunnel: [w468] -> w465
          tunnel: [w486] -> w461
          tunnel: w467 -> [w484]
          tunnel: w466 -> [w488]
          tunnel: w465 -> [_]
          tunnel: [w487] -> w460
          frame #0 {
            n181 = local read "Screen Index"() -> (w468:i32)
            n182 = case shown="0, Default" w468 {
              selector: w468 -> [_ w480]
              tunnel: w472 -> [w474 w476]
              tunnel: [w474 w478] -> w471
              tunnel: w470 -> [w473 w479]
              tunnel: [w473 w479] -> w469
              frame -1, 2 {
              }
              frame 0, Default {
                n183 = invoke on="Sub Panel" class="SubPnl" method="Remove VI"(error in=w476) -> (error out=w475:errorcluster)  [unwired: 2 in, 2 out]
                n184 = Index Array(array=w479, index=w480) -> (element=w477:refnum<vi>)
                n185 = call "if VI is running stop VI.vi"("error in (no error)"=w475, "VI in"=w477) -> ("error out"=w478:errorcluster)  [unwired: 8 in, 1 out]
              }
            }
          }
          frame #1 {
            n186 = Index Array(array=w488, index=4) -> (element=w482:refnum<vi>)
            n187 = property class="VI"(reference=w482, error in=w484) -> (error out=w483:errorcluster, "Exec.State"=w481:T5)  [unwired: 1 out]
            n188 = case shown="\"Idle\", Default" w481 {
              tunnel: w483 -> [w491 w496]
              tunnel: [w491 w493] -> w486
              tunnel: w488 -> [_ w497]
              tunnel: [7 w495] -> w487
              frame "Bad" {
                n189 = One Button Dialog(message="Manual Mode  is Running") -> ()  [unwired: 1 in, 1 out]
              }
              frame "Idle", Default {
                w495 = 2 ("index")
                n190 = local write "Screen Index"(w495) -> ()
                n191 = Index Array(array=w497, index=w495) -> (element=w498:refnum<vi>)
                n192 = call "if VI is idle run VI.vi"("error in (no error)"=w496, "VI in"=w498) -> ("error out"=w492:errorcluster, "VI out"=w494:refnum<vi>)  [unwired: 8 in]
                n193 = invoke on="Sub Panel" class="SubPnl" method="Insert VI"(error in=w492, "VI Ref"=w494) -> (error out=w493:errorcluster)  [unwired: 2 in, 3 out]
              }
            }
          }
        }
        n194 = call "Change menu button color as per screen index.vi"("error in (no error)"=w461, "Screen Index"=w460, "Array"=w462) -> ("error out"=w459:errorcluster)  [unwired: 8 in]
      }
      event "MANUAL": Value Change {
        n195 = event-data() -> ()  [unwired: 1 in, 1 out]
        n196 = invoke on="Sub Panel" class="SubPnl" method="Remove VI"(error in=w501) -> (error out=w505:errorcluster)  [unwired: 2 in, 2 out]
        n197 = flat-sequence {
          tunnel: w505 -> [w512]
          tunnel: w502 -> [w510]
          tunnel: [w511] -> w507
          tunnel: [w509] -> w506
          tunnel: [w529] -> w504
          tunnel: w507 -> [w521]
          tunnel: w506 -> [w527]
          tunnel: [w528] -> w503
          frame #0 {
            n198 = local read "Screen Index"() -> (w508:i32)
            n199 = case shown="-1, 2" w508 {
              selector: w508 -> [_ w519]
              tunnel: w512 -> [w514 w517]
              tunnel: [w514 w516] -> w511
              tunnel: w510 -> [w513 w518]
              tunnel: [w513 w518] -> w509
              frame -1, 2 {
              }
              frame 0, Default {
                n200 = Index Array(array=w518, index=w519) -> (element=w515:refnum<vi>)
                n201 = call "if VI is running stop VI.vi"("error in (no error)"=w517, "VI in"=w515) -> ("error out"=w516:errorcluster)  [unwired: 8 in, 1 out]
              }
            }
          }
          frame #1 {
            n202 = Index Array(array=w527, index=3) -> (element=w522:refnum<vi>)
            n203 = property class="VI"(reference=w522, error in=w521) -> (error out=w525:errorcluster, "Exec.State"=w524:T5)  [unwired: 1 out]
            n204 = case shown="\"Idle\", Default" w524 {
              tunnel: w525 -> [w530 w532]
              tunnel: [TRUE FALSE] -> w523
              tunnel: [w530 w532] -> w520
              frame "Idle", Default {
              }
              frame "Run top level", "Running" {
              }
            }
            n205 = case shown="True" w523 {
              tunnel: w527 -> [_ w543]
              tunnel: [w535 w542] -> w529
              tunnel: w520 -> [w535 w541]
              tunnel: [3 ("index") w537] -> w528
              frame False {
                n206 = One Button Dialog(message="Auto Cycle is Running Go to Auto Cycle and Press EXIT") -> ()  [unwired: 1 in, 1 out]
              }
              frame True {
                w537 = 4 ("index")
                n207 = Index Array(array=w543, index=w537) -> (element=w538:refnum<vi>)
                n208 = call "if VI is idle run VI.vi"("error in (no error)"=w541, "VI in"=w538) -> ("error out"=w540:errorcluster, "VI out"=w539:refnum<vi>)  [unwired: 8 in]
                n209 = local write "Screen Index"(w537) -> ()
                n210 = invoke on="Sub Panel" class="SubPnl" method="Insert VI"(error in=w540, "VI Ref"=w539) -> (error out=w542:errorcluster)  [unwired: 2 in, 3 out]
              }
            }
          }
        }
        n211 = call "Change menu button color as per screen index.vi"("error in (no error)"=w504, "Screen Index"=w503, "Array"=w500) -> ("error out"=w499:errorcluster)  [unwired: 8 in]
      }
      event "REPORT": Value Change {
        n212 = event-data() -> ()  [unwired: 1 in, 3 out]
        n213 = invoke on="Sub Panel" class="SubPnl" method="Remove VI"(error in=w544) -> (error out=w549:errorcluster)  [unwired: 2 in, 2 out]
        n214 = flat-sequence {
          tunnel: w549 -> [w558]
          tunnel: w552 -> [w555]
          tunnel: [w557] -> w551
          tunnel: [w554] -> w550
          tunnel: [w571] -> w547
          tunnel: w551 -> [w570]
          tunnel: w550 -> [w572]
          tunnel: [w566] -> w545
          frame #0 {
            n215 = local read "Screen Index"() -> (w556:i32)
            n216 = case shown="-1, 2" w556 {
              selector: w556 -> [_ w565]
              tunnel: w558 -> [w560 w563]
              tunnel: [w560 w562] -> w557
              tunnel: w555 -> [w559 w564]
              tunnel: [w559 w564] -> w554
              frame -1, 2 {
              }
              frame 0, Default {
                n217 = Index Array(array=w564, index=w565) -> (element=w561:refnum<vi>)
                n218 = call "if VI is running stop VI.vi"("error in (no error)"=w563, "VI in"=w561) -> ("error out"=w562:errorcluster)  [unwired: 8 in, 1 out]
              }
            }
          }
          frame #1 {
            w566 = 3 ("index")
            n219 = local write "Screen Index"(w566) -> ()
            n220 = Index Array(array=w572, index=w566) -> (element=w567:refnum<vi>)
            n221 = call "if VI is idle run VI.vi"("error in (no error)"=w570, "VI in"=w567) -> ("error out"=w569:errorcluster, "VI out"=w568:refnum<vi>)  [unwired: 8 in]
            n222 = invoke on="Sub Panel" class="SubPnl" method="Insert VI"(error in=w569, "VI Ref"=w568) -> (error out=w571:errorcluster)  [unwired: 2 in, 3 out]
          }
        }
        n223 = call "Change menu button color as per screen index.vi"("error in (no error)"=w547, "Screen Index"=w545, "Array"=w546) -> ("error out"=w548:errorcluster)  [unwired: 8 in]
      }
      event "andon": Value Change {
        n224 = event-data() -> ()  [unwired: 1 in, 3 out]
        n225 = invoke on="Sub Panel" class="SubPnl" method="Remove VI"(error in=w573) -> (error out=w578:errorcluster)  [unwired: 2 in, 2 out]
        n226 = flat-sequence {
          tunnel: w578 -> [w587]
          tunnel: w581 -> [w584]
          tunnel: [w586] -> w580
          tunnel: [w583] -> w579
          tunnel: [w600] -> w576
          tunnel: w580 -> [w599]
          tunnel: w579 -> [w601]
          tunnel: [w595] -> w575
          frame #0 {
            n227 = local read "Screen Index"() -> (w585:i32)
            n228 = case shown="-1, 2" w585 {
              selector: w585 -> [_ w594]
              tunnel: w587 -> [w589 w592]
              tunnel: [w589 w591] -> w586
              tunnel: w584 -> [w588 w593]
              tunnel: [w588 w593] -> w583
              frame -1, 2 {
              }
              frame 0, Default {
                n229 = Index Array(array=w593, index=w594) -> (element=w590:refnum<vi>)
                n230 = call "if VI is running stop VI.vi"("error in (no error)"=w592, "VI in"=w590) -> ("error out"=w591:errorcluster)  [unwired: 8 in, 1 out]
              }
            }
          }
          frame #1 {
            w595 = 6 ("index")
            n231 = local write "Screen Index"(w595) -> ()
            n232 = Index Array(array=w601, index=w595) -> (element=w596:refnum<vi>)
            n233 = call "if VI is idle run VI.vi"("error in (no error)"=w599, "VI in"=w596) -> ("error out"=w598:errorcluster, "VI out"=w597:refnum<vi>)  [unwired: 8 in]
            n234 = invoke on="Sub Panel" class="SubPnl" method="Insert VI"(error in=w598, "VI Ref"=w597) -> (error out=w600:errorcluster)  [unwired: 2 in, 3 out]
          }
        }
        n235 = call "Change menu button color as per screen index.vi"("error in (no error)"=w576, "Screen Index"=w575, "Array"=w574) -> ("error out"=w577:errorcluster)  [unwired: 8 in]
      }
      event "Hardware Setting": Value Change {
        n236 = event-data() -> ()  [unwired: 1 in, 3 out]
        n237 = invoke on="Sub Panel" class="SubPnl" method="Remove VI"(error in=w602) -> (error out=w607:errorcluster)  [unwired: 2 in, 2 out]
        n238 = flat-sequence {
          tunnel: w607 -> [w616]
          tunnel: w610 -> [w613]
          tunnel: [w615] -> w609
          tunnel: [w612] -> w608
          tunnel: [w629] -> w605
          tunnel: w609 -> [w628]
          tunnel: w608 -> [w630]
          tunnel: [w624] -> w604
          frame #0 {
            n239 = local read "Screen Index"() -> (w614:i32)
            n240 = case shown="-1, 2" w614 {
              selector: w614 -> [_ w623]
              tunnel: w616 -> [w618 w621]
              tunnel: [w618 w620] -> w615
              tunnel: w613 -> [w617 w622]
              tunnel: [w617 w622] -> w612
              frame -1, 2 {
              }
              frame 0, Default {
                n241 = Index Array(array=w622, index=w623) -> (element=w619:refnum<vi>)
                n242 = call "if VI is running stop VI.vi"("error in (no error)"=w621, "VI in"=w619) -> ("error out"=w620:errorcluster)  [unwired: 8 in, 1 out]
              }
            }
          }
          frame #1 {
            w624 = 4 ("index")
            n243 = local write "Screen Index"(w624) -> ()
            n244 = Index Array(array=w630, index=w624) -> (element=w625:refnum<vi>)
            n245 = call "if VI is idle run VI.vi"("error in (no error)"=w628, "VI in"=w625) -> ("error out"=w627:errorcluster, "VI out"=w626:refnum<vi>)  [unwired: 8 in]
            n246 = invoke on="Sub Panel" class="SubPnl" method="Insert VI"(error in=w627, "VI Ref"=w626) -> (error out=w629:errorcluster)  [unwired: 2 in, 3 out]
          }
        }
        n247 = call "Change menu button color as per screen index.vi"("error in (no error)"=w605, "Screen Index"=w604, "Array"=w603) -> ("error out"=w606:errorcluster)  [unwired: 8 in]
      }
      event "Shift Setting": Value Change {
        n248 = event-data() -> ()  [unwired: 1 in, 3 out]
        n249 = invoke on="Sub Panel" class="SubPnl" method="Remove VI"(error in=w631) -> (error out=w636:errorcluster)  [unwired: 2 in, 2 out]
        n250 = flat-sequence {
          tunnel: w636 -> [w645]
          tunnel: w639 -> [w642]
          tunnel: [w644] -> w638
          tunnel: [w641] -> w637
          tunnel: [w658] -> w632
          tunnel: w638 -> [w657]
          tunnel: w637 -> [w659]
          tunnel: [w653] -> w634
          frame #0 {
            n251 = local read "Screen Index"() -> (w643:i32)
            n252 = case shown="-1, 2" w643 {
              selector: w643 -> [_ w652]
              tunnel: w645 -> [w647 w650]
              tunnel: [w647 w649] -> w644
              tunnel: w642 -> [w646 w651]
              tunnel: [w646 w651] -> w641
              frame -1, 2 {
              }
              frame 0, Default {
                n253 = Index Array(array=w651, index=w652) -> (element=w648:refnum<vi>)
                n254 = call "if VI is running stop VI.vi"("error in (no error)"=w650, "VI in"=w648) -> ("error out"=w649:errorcluster)  [unwired: 8 in, 1 out]
              }
            }
          }
          frame #1 {
            w653 = 5 ("index")
            n255 = local write "Screen Index"(w653) -> ()
            n256 = Index Array(array=w659, index=w653) -> (element=w654:refnum<vi>)
            n257 = call "if VI is idle run VI.vi"("error in (no error)"=w657, "VI in"=w654) -> ("error out"=w656:errorcluster, "VI out"=w655:refnum<vi>)  [unwired: 8 in]
            n258 = invoke on="Sub Panel" class="SubPnl" method="Insert VI"(error in=w656, "VI Ref"=w655) -> (error out=w658:errorcluster)  [unwired: 2 in, 3 out]
          }
        }
        n259 = call "Change menu button color as per screen index.vi"("error in (no error)"=w632, "Screen Index"=w634, "Array"=w633) -> ("error out"=w635:errorcluster)  [unwired: 8 in]
      }
      event "Test Print": Value Change {
        n260 = event-data() -> ()  [unwired: 1 in, 3 out]
        n261 = invoke on="Sub Panel" class="SubPnl" method="Remove VI"(error in=w660) -> (error out=w665:errorcluster)  [unwired: 2 in, 2 out]
        n262 = flat-sequence {
          tunnel: w665 -> [w674]
          tunnel: w668 -> [w671]
          tunnel: [w673] -> w667
          tunnel: [w670] -> w666
          tunnel: [w687] -> w663
          tunnel: w667 -> [w686]
          tunnel: w666 -> [w688]
          tunnel: [w682] -> w662
          frame #0 {
            n263 = local read "Screen Index"() -> (w672:i32)
            n264 = case shown="-1, 2" w672 {
              selector: w672 -> [_ w681]
              tunnel: w674 -> [w676 w679]
              tunnel: [w676 w678] -> w673
              tunnel: w671 -> [w675 w680]
              tunnel: [w675 w680] -> w670
              frame -1, 2 {
              }
              frame 0, Default {
                n265 = Index Array(array=w680, index=w681) -> (element=w677:refnum<vi>)
                n266 = call "if VI is running stop VI.vi"("error in (no error)"=w679, "VI in"=w677) -> ("error out"=w678:errorcluster)  [unwired: 8 in, 1 out]
              }
            }
          }
          frame #1 {
            w682 = 9 ("index")
            n267 = local write "Screen Index"(w682) -> ()
            n268 = Index Array(array=w688, index=w682) -> (element=w683:refnum<vi>)
            n269 = call "if VI is idle run VI.vi"("error in (no error)"=w686, "VI in"=w683) -> ("error out"=w685:errorcluster, "VI out"=w684:refnum<vi>)  [unwired: 8 in]
            n270 = invoke on="Sub Panel" class="SubPnl" method="Insert VI"(error in=w685, "VI Ref"=w684) -> (error out=w687:errorcluster)  [unwired: 2 in, 3 out]
          }
        }
        n271 = call "Change menu button color as per screen index.vi"("error in (no error)"=w663, "Screen Index"=w662, "Array"=w661) -> ("error out"=w664:errorcluster)  [unwired: 8 in]
      }
      event "Home": Value Change {
        n272 = event-data() -> ()  [unwired: 1 in, 3 out]
        n273 = invoke on="Sub Panel" class="SubPnl" method="Remove VI"(error in=w689) -> (error out=w692:errorcluster)  [unwired: 2 in, 2 out]
        n274 = call "Change menu button color as per screen index.vi"("error in (no error)"=w692, "Screen Index"=-1, "Array"=w690) -> ("error out"=w691:errorcluster)  [unwired: 8 in]
      }
      event "EXIT": Value Change {
        n275 = event-data() -> ()  [unwired: 1 in, 1 out]
        n276 = Index Array(array=w698, index=2) -> (element=w704:refnum<vi>)
        n277 = Build Array(w704) -> (w703:refnum<vi>[])
        n278 = for {
          tunnel: w698 -> [w727]
          tunnel: [w726] -> w706 mode=indexing
          shift-right: [w725] -> w700
          shift-left: w705 -> [w724]
          tunnel: w703 -> [w723] mode=indexing
          n279 = property class="VI"(reference=w723, error in=w724) -> (error out=w729:errorcluster, "Exec.State"=w728:T5)  [unwired: 1 out]
          n280 = case shown="\"Run top level\", \"Running\"" w728 {
            tunnel: w729 -> [w730 w732]
            tunnel: w727 -> [_ _]
            tunnel: [TRUE FALSE] -> w726
            tunnel: [w730 w732] -> w725
            frame "Idle", Default {
            }
            frame "Run top level", "Running" {
            }
          }
        }
        n281 = And Array Elements(Boolean array=w706) -> (logical AND=w702:bool)
        n282 = case shown="False" w702 {
          tunnel: [FALSE TRUE] -> w697
          tunnel: w700 -> [w711 w715]
          tunnel: [w711 w714] -> w699
          tunnel: w698 -> [_ w713]
          frame False {
            n283 = One Button Dialog(message="Auto Cycle  is Running") -> ()  [unwired: 1 in, 1 out]
          }
          frame True {
            n284 = invoke on="Sub Panel" class="SubPnl" method="Remove VI"(error in=w715) -> (error out=w716:errorcluster)  [unwired: 2 in, 2 out]
            n285 = for {
              shift-right: [w722] -> w714
              shift-left: w716 -> [w721]
              tunnel: w713 -> [w717] mode=indexing
              n286 = call "if VI is running stop VI.vi"("error in (no error)"=w721, "VI in"=w717) -> ("error out"=w720:errorcluster, "VI out"=w719:refnum<vi>)  [unwired: 8 in]
              n287 = call <vilib>:"Clear Errors.vi"("error in (no error)"=w720) -> ("error out"=w718:errorcluster)  [unwired: 5 in, 1 out]
              n288 = Close Reference(reference=w719, error in (no error)=w718) -> (error out=w722:errorcluster)
            }
          }
        }
        n289 = global write "DATA LOG.vi" "Auto Cycle On"(FALSE) -> ()
        n290 = call "Change menu button color as per screen index.vi"("error in (no error)"=w699, "Screen Index"=-1, "Array"=w701) -> ("error out"=w696:errorcluster)  [unwired: 8 in]
      }
      event "Remove": Value Change {
        n291 = event-data() -> ()  [unwired: 1 in, 1 out]
        n292 = invoke on="Sub Panel" class="SubPnl" method="Remove VI"(error in=w734) -> (error out=w736:errorcluster)  [unwired: 2 in, 2 out]
        n293 = call "Change menu button color as per screen index.vi"("error in (no error)"=w736, "Screen Index"=-1, "Array"=w735) -> ("error out"=w737:errorcluster)  [unwired: 8 in]
      }
      event Timeout {
        n294 = event-data() -> ()  [unwired: 1 in, 1 out]
        n295 = global read "Global 1.vi" "BARCODE RECIPE"() -> (w749:string)
        n296 = global read "Global 1.vi" "MODEL SELECTION"() -> (w750:bool)
        n297 = global read "Login Details.vi" "User Name"() -> (→"user name":string)
        n298 = Format Date/Time String(time format string (%c)="%d/ %m/ %Y\n%H:%M:%S") -> (date/time string=→"datetime":string)  [unwired: 2 in]
        n299 = Empty String/Path?(string/path=w749) -> (empty?=w748:bool)
        n300 = Or(x="Check 2", y=w750) -> (x .or. y?=w754:bool)
        n301 = global read "Global 1.vi" "REMOVE VI"() -> (w751:bool)
        n302 = case shown="True" w754 {
          tunnel: w752 -> [w782 w787]
          tunnel: [w782 w786] -> w741
          tunnel: w748 -> [_ w784]
          frame False {
          }
          frame True {
            n303 = flat-sequence {
              tunnel: w787 -> [w791]
              tunnel: [w789] -> w785
              tunnel: w784 -> [w788]
              tunnel: [w788] -> w783
              tunnel: [w794] -> w786
              tunnel: w785 -> [w795]
              tunnel: w783 -> [w793]
              frame #0 {
                n304 = invoke on="Sub Panel" class="SubPnl" method="Remove VI"(error in=w791) -> (error out=w789:errorcluster)  [unwired: 2 in, 2 out]
                n305 = global write "Global 1.vi" "MODEL SELECTION"(FALSE ("remove_VI")) -> ()
                n306 = local write "Check 2"(FALSE ("Check")) -> ()
              }
              frame #1 {
                n307 = case shown="False" w793 {
                  tunnel: w795 -> [w797 w799]
                  tunnel: [w796 w799] -> w794
                  frame False {
                    n308 = property on="auto" class="Bool (strict)"(error in=w797, "Val(Sgnl)"=TRUE ("Value (Signaling)")) -> (error out=w796:errorcluster)  [unwired: 1 in, 1 out]
                  }
                  frame True {
                  }
                }
              }
            }
          }
        }
        n309 = Or(x="Check", y=w751) -> (x .or. y?=w779:bool)
        n310 = case shown="False" w779 {
          selector: w779 -> [_ w814]
          frame False {
          }
          frame True {
            n311 = global write "Global 1.vi" "REMOVE VI"(FALSE ("remove_VI")) -> ()
            n312 = property on="Remove" class="Bool (strict)"("Val(Sgnl)"=w814) -> ()  [unwired: 2 in, 2 out]
            n313 = local write "Check"(FALSE ("Check")) -> ()
          }
        }
        n314 = global read "Login Details.vi" "Authority"() -> (w775:T2)
        n315 = Unbundle By Name(w775) -> ("SCREEN 2"=w773:bool, "SCREEN 3"=w772:bool, "SCREEN 4"=w771:bool, "SCREEN 5"=w770:bool, "SCREEN 6"=w769:bool, "SCREEN 7"=w768:bool, "SCREEN 8"=w767:bool, "SCREEN 9"=w766:bool, "SCREEN 10"=w765:bool, "SCREEN 11"=w764:bool, "SCREEN 12"=w763:bool, "SCREEN 13"=w762:bool, "SCREEN 14"=w761:bool, "SCREEN 15"=w760:bool, "SCREEN 16"=w759:bool, "SCREEN 17"=w758:bool, "SCREEN 18"=w757:bool, "SCREEN 19"=w756:bool, "SCREEN 20"=w755:bool)  [unwired: 1 out]
        n316 = control-ref of="Hardware Setting"() -> (w744:refnum<vi>)
        n317 = control-ref of="Shift Setting"() -> (w743:refnum<vi>)
        n318 = control-ref of="REPORT"() -> (w745:refnum<vi>)
        n319 = control-ref of="USER MANGMENT"() -> (w747:refnum<vi>)
        n320 = control-ref of="AUTO MODE"() -> (w746:refnum<vi>)
        n321 = Build Array(w747, w746, w745, w744, w743) -> (w742:refnum<vi>[])
        n322 = Build Array(w773, w772, w771, w770, w769, w768, w767, w766, w765, w764, w763, w762, w761, w760, w759, w758, w757, w756, w755) -> (w774:bool[])
        n323 = for {
          tunnel: w774 -> [w802] mode=indexing
          tunnel: w742 -> [w803] mode=indexing
          tunnel: w741 -> [w801]
          tunnel: [w800] -> w740
          n324 = case shown="True" w802 {
            tunnel: w803 -> [w806 w810]
            tunnel: w801 -> [w805 w809]
            tunnel: [w804 w808] -> w800
            frame True {
              n325 = property class="Bool"(reference=w806, error in=w805, "DisabledEnum"=T3."Enabled" ("Disabled")) -> (error out=w804:errorcluster)  [unwired: 1 out]
            }
            frame False {
              n326 = property class="Bool"(reference=w810, error in=w809, "DisabledEnum"=T3."Disabled and Grayed Out" ("Disabled")) -> (error out=w808:errorcluster)  [unwired: 1 out]
            }
          }
        }
      }
    }
  }
  n327 = disable-structure shown="Disabled" {
    disable-tunnel: w3 -> [w815 _]
    frame Disabled {
      n328 = Quit LabVIEW(quit? (T)=w815) -> ()
    }
    frame Enabled {
    }
  }
  n329 = call <vilib>:"Clear Errors.vi"("error in (no error)"=w22) -> ("error out"=w12:errorcluster)  [unwired: 5 in, 1 out]
  n330 = call "PADMINI_STOP_ALL.vi"("Enum"=enum16{"Read", "Write"}."Write", "error in (no error)"=w12, "Boolean"=TRUE) -> ("error out"=w9:errorcluster)  [unwired: 7 in, 1 out]
  n331 = call <vilib>:"Clear Errors.vi"("error in (no error)"=w9) -> ("error out"=w35:errorcluster)  [unwired: 5 in, 1 out]
  n332 = property class="App"(error in=w35) -> (error out=w36:errorcluster, "App.Kind"=w37:T6)  [unwired: 1 in, 1 out]
  n333 = case shown="\"Run Time System\"" w37 {
    tunnel: w36 -> [w816 w818]
    tunnel: [w816 w817] -> w34
    frame Default {
    }
    frame "Run Time System" {
      n334 = invoke class="VI" method="FP.Close"(error in=w818) -> (error out=w817:errorcluster)  [unwired: 2 in, 2 out]
    }
  }
  "error out 2" <- w34
